vi "readFromXML.vi"(8 "error in (no error)":errorcluster, 10 "XML in":string="<AOSPointingOffset>\n  <commandID>1234</commandID>\n  <tcsErrorResponse>\n   <status>true</status>\n    <code>0</code>\n    <source/>\n  </tcsErrorResponse>\n\t\t<xCorrection_arcsec>66</xCorrection_arcsec>\n\t\t<yCorrection_arcsec>55</yCorrection_arcsec>\n</AOSPointingOffset>", 11 "TCSActiveOpticsCommand in":refnum<class "TCSActiveOpticsCommand.lvclass">) -> (0 "error out":errorcluster, 3 "TCSActiveOpticsCommand out":refnum<class "TCSActiveOpticsCommand.lvclass">)   [LabVIEW 2014, in "TCSDataDefinitions.lvlib" / "TCSActiveOpticsCommand.lvlib" / "TCSActiveOpticsCommand.lvclass"]
uses:
  TCSActiveOpticsCommand.lvclass
  TCSCommand/TCSCommand/TCSCommand.lvclass
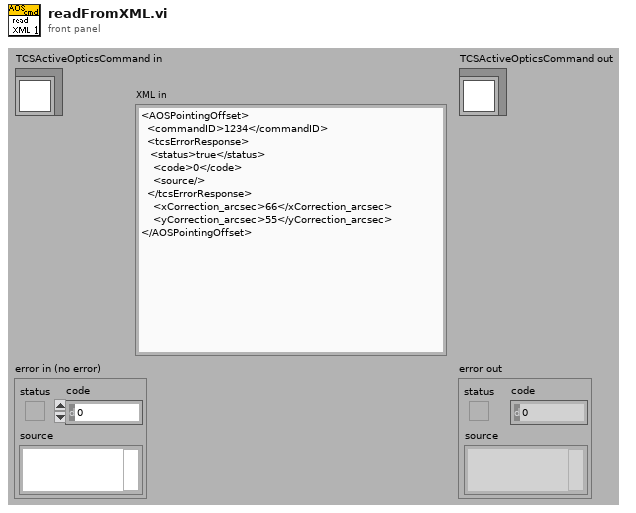
[diagram p1: front panel]
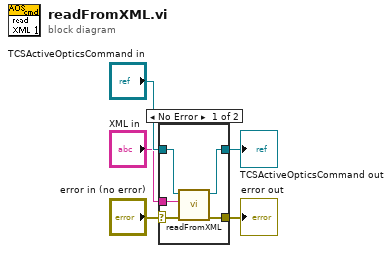
[diagram p0: block diagram]
diagram:
  n1 = case shown="No Error" "error in (no error)" {
    selector: "error in (no error)" -> [w7 w12]
    tunnel: [w6 w12] -> w4
    tunnel: [w8 w11] -> w2
    tunnel: "TCSActiveOpticsCommand in" -> [w9 w11]
    tunnel: "XML in" -> [w10 _]
    frame No Error {
      n2 = call-parent "readFromXML.vi"("error in (no error)"=w7, "XML in"=w10, "TCSCommand in"=w9) -> ("error out"=w6:errorcluster, "TCSCommand out"=w8:refnum<class "TCSActiveOpticsCommand.lvclass">)  [unwired: 7 in]
    }
    frame Error {
    }
  }
  "error out" <- w4
  "TCSActiveOpticsCommand out" <- w2
